vi "Set Capacitance.vi"(8 "error in (no error)":errorcluster, 9 "Channel":i32, 10 "Capacitance (pF)":dbl, 11 "Instrument.CBridge in":refnum<class "Instrument.CBridge.lvclass">) -> (0 "error out":errorcluster, 3 "Instrument.CBridge out":refnum<class "Instrument.CBridge.lvclass">)   [LabVIEW 2016, in "Instrument.CBridge.lvclass"]
uses:
  Instrument.CBridge.lvclass
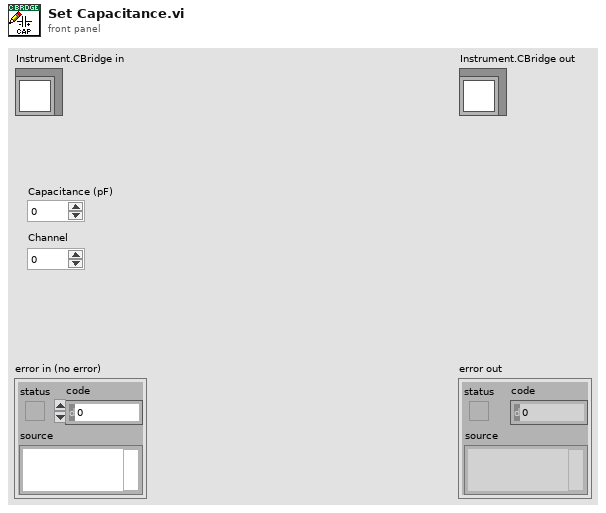
[diagram p1: front panel]
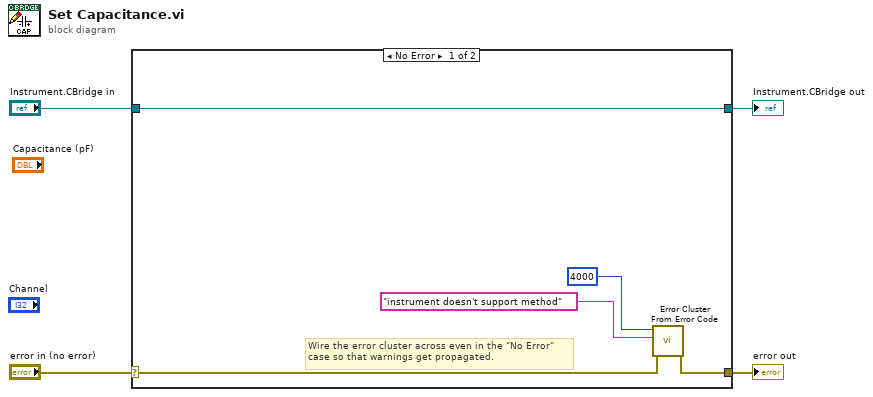
[diagram p0: block diagram]
diagram:
  n1 = case shown="No Error" "error in (no error)" {
    selector: "error in (no error)" -> [w6 w11]
    tunnel: [w5 w11] -> w3
    tunnel: [w9 w10] -> w1
    tunnel: "Instrument.CBridge in" -> [w9 w10]
    frame No Error {
      # "Wire the error cluster across even in the \"No Error\"\ncase so that warnings get propagated."
      n2 = call <vilib>:"Error Cluster From Error Code.vi"("error in (no error)"=w6, "error message (\"\")"="instrument doesn't support method" ("error message (\"\")"), "error code (0)"=4000) -> ("error out"=w5:errorcluster)  [unwired: 6 in]
    }
    frame Error {
    }
  }
  "error out" <- w3
  "Instrument.CBridge out" <- w1
